vi "PolishVisionV4.vi"() -> (0 "Status":bool, 1 "Source CODE Robot":string, 3 "WorkPiece In Process":T1(plugin-control))   [LabVIEW 2015]
uses:
  <vilib>/userdefined/High Color/IMAQdx.ctl
  <vilib>/vision/driver/NI_Vision_Acquisition_Software.lvlib
  <vilib>/vision/NI_Vision_Development_Module.lvlib
panel:
  out "Edge Right Side":cluster{cluster{"Xrn":dbl, "Yrn":dbl}}[][](array[cluster])
  out "Edge Lefe Side":cluster{cluster{"Xln":dbl, "Yln":dbl}}[][](array[cluster])
  in  "WP Length":sgl=177.0
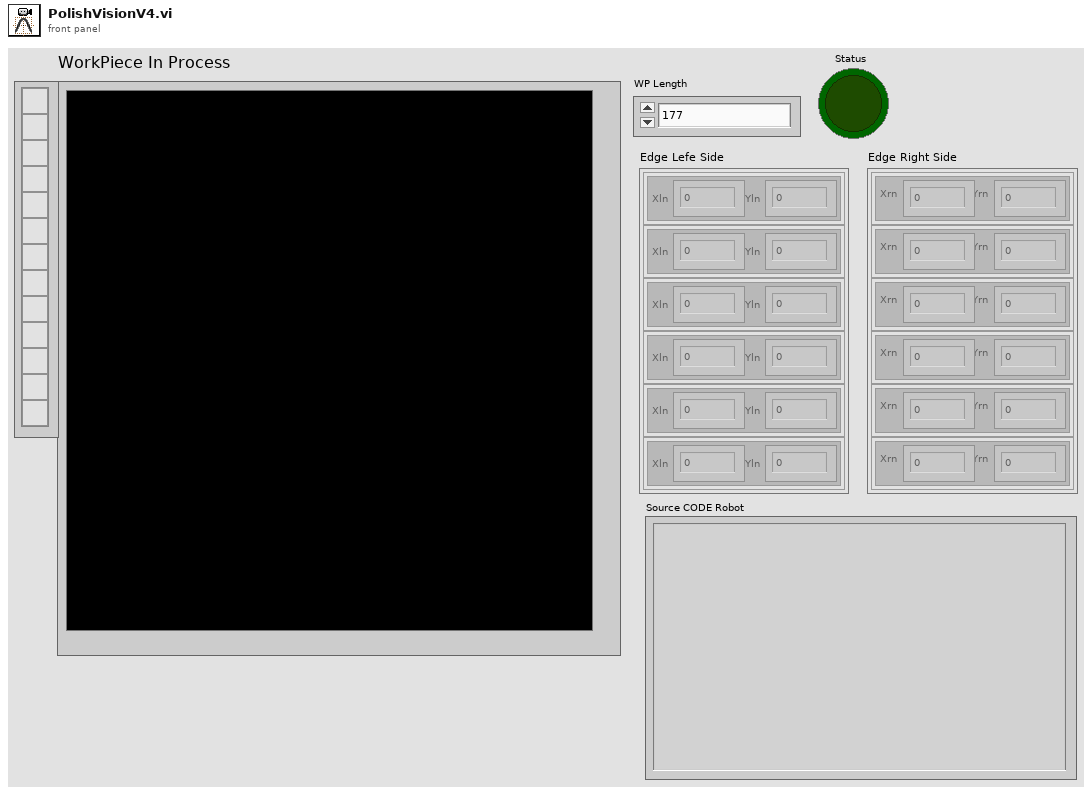
[diagram p1: front panel]
types:
  T1 = typedef "IMAQ Image.ctl" = refnum<image>
  T2 = typedef "IMAQdx.ctl" = refnum<k21>
  T3 = typedef "Image Type" = u32
  T4 = cluster{"Number of Matches Requested":i32, "Minimum Match Score":sgl, "Angle Ranges":cluster{"Start Angle":sgl, "End Angle":sgl}[]}
  T5 = cluster{"Global Rectangle":i32[], "Contours":cluster{"ID":enum32{"External", "Internal"}, "Type":u32, "Coordinates":i32[]}[]}
  T6 = cluster{"Origin Pixel":cluster{"X":sgl, "Y":sgl}, "X Axis Pixel":cluster{"X":sgl, "Y":sgl}, "Axis Reference":u32}
  T7 = cluster{"Position":cluster{"x":sgl, "y":sgl}, "Angle":sgl, "Scale":sgl, "Score":sgl, "Bounding Box":cluster{"x":sgl, "y":sgl}[]}[]
  T8 = cluster{"Feature":u32, "Points IDs":cluster{"GUID":string, "Index":i32}[]}[]
  T9 = cluster{"Matches (pixel)[0]":cluster{"Position":cluster{"x":sgl, "y":sgl}, "Angle":sgl, "Scale":sgl, "Score":sgl, "Bounding Box":cluster{"x":sgl, "y":sgl}[]}, "Matches (pixel)[1]":cluster{"Position":cluster{"x":sgl, "y":sgl}, "Angle":sgl, "Scale":sgl, "Score":sgl, "Bounding Box":cluster{"x":sgl, "y":sgl}[]}, "Matches (pixel)[2]":cluster{"Position":cluster{"x":sgl, "y":sgl}, "Angle":sgl, "Scale":sgl, "Score":sgl, "Bounding Box":cluster{"x":sgl, "y":sgl}[]}, "Matches (pixel)[3]":cluster{"Position":cluster{"x":sgl, "y":sgl}, "Angle":sgl, "Scale":sgl, "Score":sgl, "Bounding Box":cluster{"x":sgl, "y":sgl}[]}, "Matches (pixel)[4]":cluster{"Position":cluster{"x":sgl, "y":sgl}, "Angle":sgl, "Scale":sgl, "Score":sgl, "Bounding Box":cluster{"x":sgl, "y":sgl}[]}, "Matches (pixel)[5]":cluster{"Position":cluster{"x":sgl, "y":sgl}, "Angle":sgl, "Scale":sgl, "Score":sgl, "Bounding Box":cluster{"x":sgl, "y":sgl}[]}, "Matches (pixel)[6]":cluster{"Position":cluster{"x":sgl, "y":sgl}, "Angle":sgl, "Scale":sgl, "Score":sgl, "Bounding Box":cluster{"x":sgl, "y":sgl}[]}, "Matches (pixel)[7]":cluster{"Position":cluster{"x":sgl, "y":sgl}, "Angle":sgl, "Scale":sgl, "Score":sgl, "Bounding Box":cluster{"x":sgl, "y":sgl}[]}, "Matches (pixel)[8]":cluster{"Position":cluster{"x":sgl, "y":sgl}, "Angle":sgl, "Scale":sgl, "Score":sgl, "Bounding Box":cluster{"x":sgl, "y":sgl}[]}}
  T10 = cluster{"Results (Pixels)[0]":sgl, "Results (Pixels)[1]":sgl, "Results (Pixels)[2]":sgl, "Results (Pixels)[3]":sgl, "Results (Pixels)[4]":sgl, "Results (Pixels)[5]":sgl, "Results (Pixels)[6]":sgl, "Results (Pixels)[7]":sgl, "Results (Pixels)[8]":sgl}
  T11 = cluster{"Results (Pixels)[0]":sgl, "Results (Pixels)[1]":sgl}
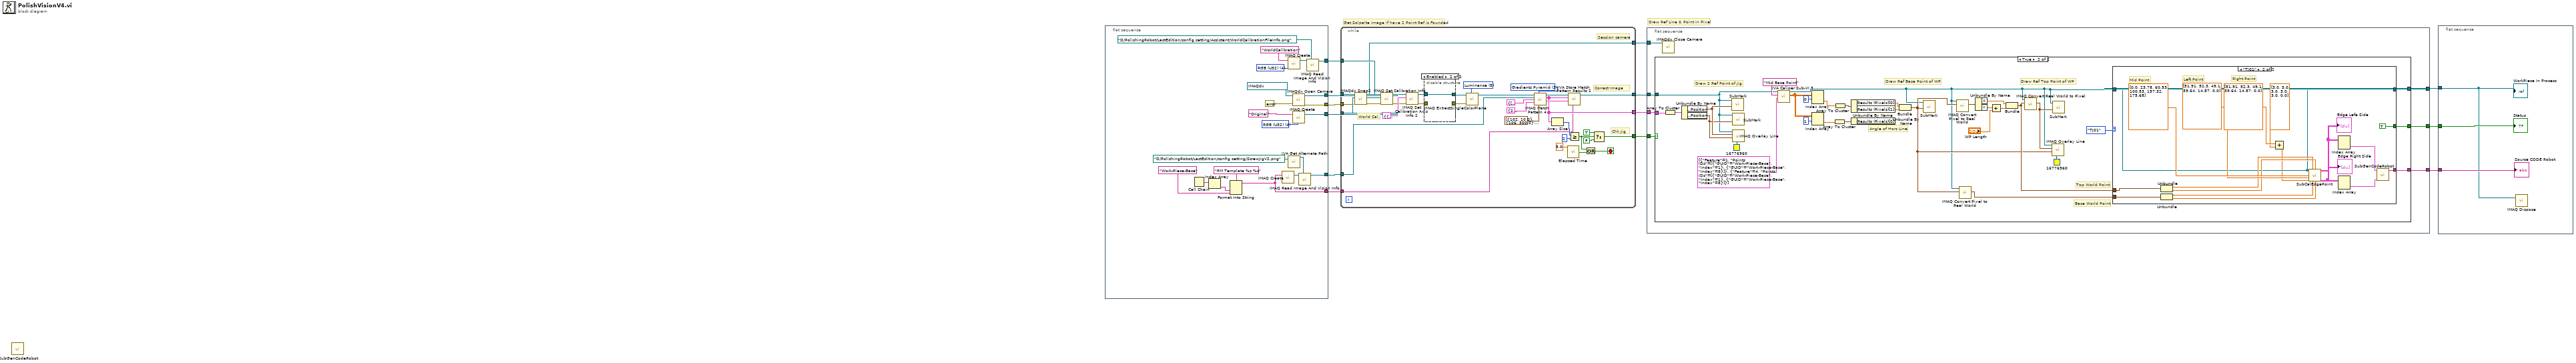
[diagram p0: block diagram]
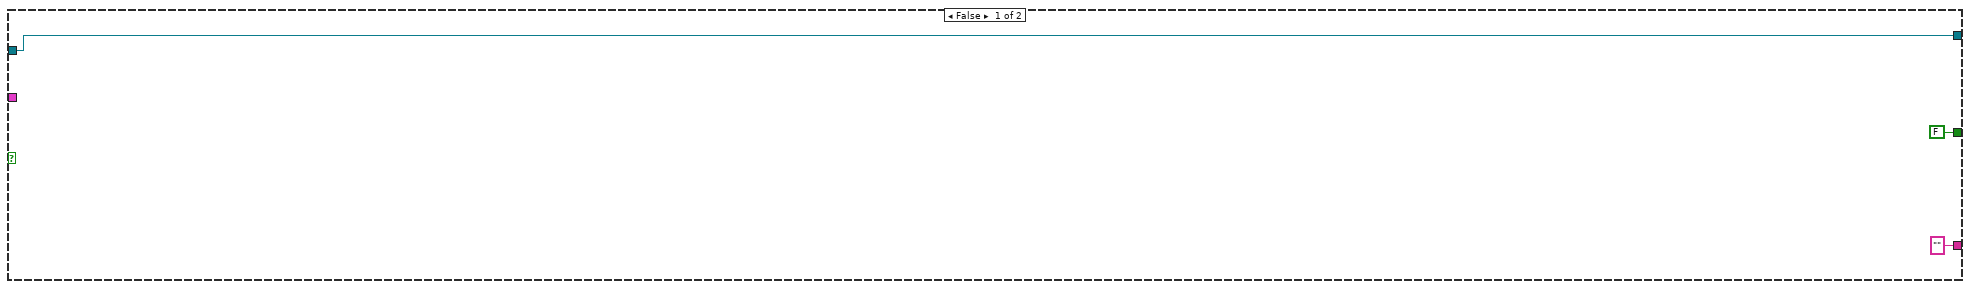
[diagram p2: hidden frame]
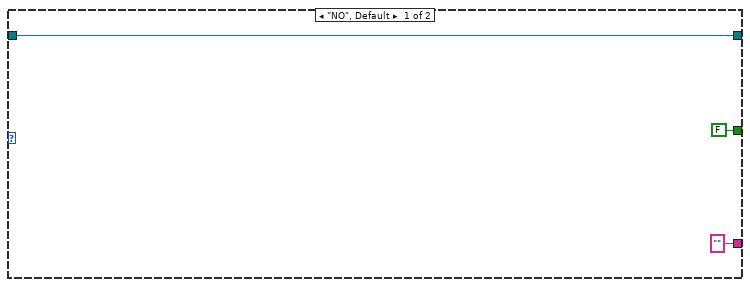
[diagram p3: hidden frame]
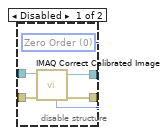
[diagram p4: hidden frame]
diagram:
  # "Draw Ref Line & Point in Pixel"
  # "Get Solpalte Image if have 2 Point Ref is Founded"
  n1 = call "SubGenCodeRobot.vi"() -> ()  [unwired: 11 in, 1 out]
  n2 = flat-sequence {
    tunnel: [w31] -> w13
    tunnel: [w30] -> w12
    tunnel: [w29] -> w10
    tunnel: [w23] -> w11
    tunnel: [w19] -> w9
    tunnel: [w14] -> w5
    frame #0 {
      w27 = T3 4 items=["Grayscale (U8)", "Grayscale (I16)", "Grayscale (SGL)", "Complex (CSG)", "RGB (U32)", "HSL (U32)", "RGB (U64)", "Grayscale (U16)"] ("Image Type")
      w32 = T3 4 items=["Grayscale (U8)", "Grayscale (I16)", "Grayscale (SGL)", "Complex (CSG)", "RGB (U32)", "HSL (U32)", "RGB (U64)", "Grayscale (U16)"] ("Image Type")
      n3 = Call Chain() -> (call chain=w17:string[])
      n4 = Index Array(array=w17) -> (element=w16:string)  [unwired: 1 in]
      n5 = Format Into String(format string="PM Template %s %s" ("Image Name"), w16, "Work-Piece-Base" ("Image Name")) -> (resulting string=w14:string)  [unwired: 2 in, 1 out]
      n6 = call "IMAQ Create"("Image Name"=w14) -> ("New Image"=w22:T1)  [unwired: 3 in, 2 out]
      n7 = call <vilib>:"IVA Get Alternate Path.vi"("Path In"=path "D:/PolishingRobot/LastEdition/config setting/ScrewJigV2.png" ("Template File Path")) -> ("Path Out"=w20:path)  [unwired: 10 out]
      n8 = call "IMAQ Create"("Image Name"="WorldCalibration", "Image Type"=w27) -> ("New Image"=w26:T1)  [unwired: 2 in, 2 out]
      n9 = call <vilib>:"IMAQdx Open Camera.vi"("error in"=errorcluster {"status"=FALSE, "code"=0, "source"=""}, "Session In"=T2 "RobotPolishCAM") -> ("error out"=w29:errorcluster, "Session Out"=w31:T2)  [unwired: 8 in]
      n10 = call "IMAQ Create"("Image Name"="Original", "Image Type"=w32) -> ("New Image"=w30:T1)  [unwired: 3 in, 1 out]
      n11 = call "IMAQ Read Image And Vision Info"("File Path"=w20, "Image"=w22) -> ("Image Out"=w19:T1)  [unwired: 2 in, 7 out]
      n12 = call "IMAQ Read Image And Vision Info"("File Path"=path "D:/PolishingRobot/LastEdition/config setting/Assistant/WorldCalibrationFileInfo.png", "Image"=w26) -> ("Image Out"=w23:T1)  [unwired: 2 in, 7 out]
    }
  }
  n13 = while {
    tunnel: w13 -> [w69]
    tunnel: w12 -> [w68]
    tunnel: w11 -> [w58]
    tunnel: w10 -> [w57]
    tunnel: [w55] -> w8
    tunnel: w9 -> [w47]
    tunnel: [w43] -> w6
    tunnel: [w42] -> w7
    tunnel: w5 -> [w38]
    tunnel: [w36] -> w4
    stop <- w60 stop-if-true
    w54 = 3 items=["All", "Low Discrepancy Sampling", "Grayscale Value Pyramid", "Gradients Pyramid"] ("Algorithm")
    w67 = 5 items=["Red", "Green", "Blue", "Hue", "Saturation", "Luminance", "Value", "Intensity"] ("Color Plane")
    # "Chk Jig"
    # "Correct Image"
    # "Session camera"
    # "World Cal."
    n14 = call <vilib>:"IMAQdx Snap2.vi"("error in"=w57, "Image In"=w68, "Session In"=w69) -> ("error out"=w56:errorcluster, "Image Out"=w59:T1, "Session Out"=w55:T2)  [unwired: 6 in]
    n15 = call "IMAQ Set Calibration Info"("error in (no error)"=w56, "Image Dst"=w59, "Image Src"=w58) -> ("error out"=w41:errorcluster, "Calibrated Image"=w65:T1)  [unwired: 1 in, 6 out]
    n16 = call-poly "IMAQ Set Calibration Axis Info 2"("error in (no error)"=w41, "Calibration Axis Info"=T6 {"Origin Pixel"={"X"=1113.64, "Y"=2715.63}, "X Axis Pixel"={"X"=1115.59, "Y"=2715.63}, "Axis Reference"=0}, "Calibration Template Image In"=w65) -> ("error out"=w40:errorcluster, "Calibration Template Image Out"=w64:T1)  [unwired: 7 out]
    n17 = disable-structure shown="Enabled" {
      disable-tunnel: w64 -> [w73 w75]
      disable-tunnel: [w72 w75] -> w63
      disable-tunnel: w40 -> [w71 _]
      disable-tunnel: [w70 _] -> w39
      frame Disabled {
        w74 = u32 0 items=["Zero Order", "Bi-Linear", "Quadratic", "Cubic Spline"] ("Interpolation Type")
        n18 = call "IMAQ Correct Calibrated Image"("Interpolation Type"=w74, "error in (no error)"=w71, "Image Src"=w73) -> ("error out"=w70:errorcluster, "Corrected Image"=w72:T1)  [unwired: 4 in, 3 out]
      }
      frame Enabled {
      }
    }
    n19 = call "IMAQ ExtractSingleColorPlane"("Color Plane"=w67, "error in (no error)"=w39, "Image Src"=w63) -> ("Image Dst Out"=w48:T1)  [unwired: 7 in, 1 out]
    n20 = call "IMAQ Match Pattern 4"("Image"=w48, "Algorithm"=w54, "Template Image"=w47, "ROI Descriptor"=T5 {"Global Rectangle"=[500, 650, 1500, 800], "Contours"=[{"ID"=enum."External", "Type"=12, "Coordinates"=[500, 650, 1500, 800, 0]}]}, "Parameters"=T4 {"Number of Matches Requested"=2, "Minimum Match Score"=500.0, "Angle Ranges"=[]}, "Advanced Options"=cluster{"Item":u16, "Value":dbl}[] [{"Item"=102, "Value"=10.0}, {"Item"=106, "Value"=300.0}, {"Item"=107, "Value"=0.0}, {"Item"=108, "Value"=6.0}, {"Item"=109, "Value"=1.0}, {"Item"=111, "Value"=20.0}, {"Item"=112, "Value"=10.0}, {"Item"=113, "Value"=20.0}, {"Item"=103, "Value"=1.0}, {"Item"=100, "Value"=1.0}]) -> ("Image (duplicate)"=w37:T1, "Matches (pixel)"=w42:T7, "Matches (real-world)"=w35:T7)  [unwired: 5 in, 2 out]
    n21 = Array Size(array=w42) -> (size(s)=w49:i32)
    n22 = call "Elapsed Time"("Time Target (s)"=5.0) -> ("Time has Elapsed"=w61:bool)  [unwired: 11 in, 7 out]
    n23 = call <vilib>:"IVA Store Match Pattern Results 2.vi"("Step Name"=w38, "Matches (real-world)"=w35, "Matches (pixel)"=w42, "Image in"=w37) -> ("Image dup"=w36:T1)  [unwired: 2 in, 5 out]
    n24 = Greater Or Equal?(x=w49, y=2) -> (x >= y?=w46:bool)
    n25 = Or(x=w46, y=w61) -> (x .or. y?=w60:bool)
    n26 = Select(t=TRUE, s=w46, f=FALSE) -> (s? t:f=w43:bool)
  }
  n27 = flat-sequence {
    tunnel: w8 -> [w82]
    tunnel: w7 -> [w81]
    tunnel: w6 -> [w80]
    tunnel: w4 -> [w79]
    tunnel: [w78] -> w3
    tunnel: [w77] -> w2
    tunnel: [w76] -> w1
    frame #0 {
      n28 = case shown="True" w80 {
        tunnel: w81 -> [_ w113]
        tunnel: w79 -> [w85 w105]
        tunnel: [w85 w88] -> w78
        tunnel: ["" ("Source CODE Robot") w87] -> w77
        tunnel: [FALSE w86] -> w76
        frame False {
        }
        frame True {
          # "Base World Point"
          # "Top World Point"
          # "Draw Ref Top Point of WP"
          # "Angle of Horz Line"
          # "Draw Ref Base Point of WP"
          # "Draw 2 Ref Point of Jig"
          n29 = Array To Cluster(array=w113) -> (cluster=w117:T9)
          n30 = Unbundle By Name(w117) -> ("Matches (pixel)[0].Position"=w115:cluster{"x":sgl, "y":sgl}, "Matches (pixel)[1].Position"=w114:cluster{"x":sgl, "y":sgl})
          n31 = call "SubMark.vi"("Refnum in"=w105, "Position Pixel"=w115) -> ()  [unwired: 8 in]
          n32 = call "SubMark.vi"("Refnum in"=w105, "Position Pixel"=w114) -> ()  [unwired: 8 in]
          n33 = call "IMAQ Overlay Line"("Color"=u32 16776960, "End Point"=w114, "Start Point"=w115, "Image"=w105) -> ()  [unwired: 6 in, 2 out]
          n34 = call <vilib>:"IVA Caliper Sub-VI 3.vi"("Parameters"=T8 [{"Feature"=1, "Points IDs"=[{"GUID"="Work-Piece-Base", "Index"=1}, {"GUID"="Work-Piece-Base", "Index"=8}]}, {"Feature"=4, "Points IDs"=[{"GUID"="Work-Piece-Base", "Index"=1}, {"GUID"="Work-Piece-Base", "Index"=8}]}], "Step Name"="Mid Base Point", "Image In"=w105) -> ("Results (Pixels)"=w103:sgl[][], "Image Out"=w90:T1)  [unwired: 2 in, 5 out]
          n35 = Index Array(array=w103, index (row)=0) -> (element=w110:sgl[])  [unwired: 1 in]
          n36 = Index Array(array=w103, index (row)=1) -> (element=w102:sgl[])  [unwired: 1 in]
          n37 = Array To Cluster(array=w102) -> (cluster=w101:T10)
          n38 = Array To Cluster(array=w110) -> (cluster=w108:T10)
          n39 = Unbundle By Name(w108) -> ("Results (Pixels)[0]"=w107:sgl, "Results (Pixels)[1]"=w106:sgl)
          n40 = Unbundle By Name(w101) -> ()  [unwired: 1 out]
          n41 = Bundle("Results (Pixels)[0]"=w107, "Results (Pixels)[1]"=w106) -> (w91:T11)  [unwired: 1 in]
          n42 = call "SubMark.vi"("Refnum in"=w90, "Position Pixel"=w91) -> ()  [unwired: 8 in]
          n43 = call "IMAQ Convert Pixel to Real World"("Pixel Coordinates"=w91, "Calibrated Image"=w90) -> ("Real World Coordinates"=w98:cluster{"X":sgl, "Y":sgl})  [unwired: 4 in, 5 out]
          n44 = call "IMAQ Convert Pixel to Real World"("Pixel Coordinates"=w91, "Calibrated Image"=w90) -> ("Real World Coordinates"=w89:cluster{"X":sgl, "Y":sgl})  [unwired: 4 in, 5 out]
          n45 = Unbundle By Name(w98) -> ("X"=w96:sgl, "Y"=w99:sgl)
          n46 = Add(x=w99, y="WP Length") -> (x+y=w97:sgl)
          n47 = Bundle("X"=w96, w97) -> (w92:cluster{"X":sgl, sgl})  [unwired: 1 in]
          n48 = call "IMAQ Convert Real World to Pixel"("Real World Coordinates"=w92, "Calibrated Image"=w90) -> ("Pixel Coordinates"=w95:cluster{"X":sgl, "Y":sgl})  [unwired: 4 in, 5 out]
          n49 = call "IMAQ Overlay Line"("Color"=u32 16776960, "End Point"=w91, "Start Point"=w95, "Image"=w90) -> ()  [unwired: 6 in, 2 out]
          n50 = call "SubMark.vi"("Refnum in"=w90, "Position Pixel"=w95) -> ()  [unwired: 8 in]
          n51 = case shown="\"TJ01\"" enum16{"NO", "TJ02", "TJ01"}."TJ01" {
            tunnel: w90 -> [w120 w130]
            tunnel: w92 -> [_ w135]
            tunnel: w89 -> [_ w136]
            tunnel: [w120 w130] -> w88
            tunnel: ["" ("Source CODE Robot") w122] -> w87
            tunnel: [FALSE TRUE] -> w86
            frame "NO", Default {
            }
            frame "TJ01" {
              # "Right Point"
              # "Left Point"
              # "Mid Point"
              n52 = Unbundle(w135) -> ("X"=w134:sgl, w133:sgl)
              n53 = Unbundle(w136) -> ("X"=w132:sgl, "Y"=w131:sgl)
              n54 = Add(x=dbl[] [51.91, 52.3, 49.1, 39.64, 14.87, 0.0] ("Mid Point"), y=dbl[] [3.0, 3.0, 3.0, 3.0, 3.0, 0.0]) -> (x+y=w127:dbl[])
              n55 = call "SubCalEdgePoint.vi"("Image dup"=w130, "Mid Point Top World X"=w134, "Mid Point Top World Y"=w133, "Mid Point"=dbl[] [0.0, 23.78, 60.53, 100.53, 157.32, 175.68], "Left Point"=dbl[] [51.91, 52.3, 49.1, 39.64, 14.87, 0.0] ("Mid Point"), "Right Point"=w127, "Mid Point Base World X"=w132, "Mid Point Base World Y"=w131) -> ("Edge Lefe Side"=w126:cluster{cluster{"Xln":dbl, "Yln":dbl}}[][], "Edge Right Side"=w123:cluster{cluster{"Xrn":dbl, "Yrn":dbl}}[][])  [unwired: 6 in]
              "Edge Lefe Side" <- w126
              "Edge Right Side" <- w123
              n56 = Index Array(array=w126) -> (element=w125:cluster{cluster{"Xln":dbl, "Yln":dbl}}[])  [unwired: 2 in]
              n57 = Index Array(array=w123) -> (element=w124:cluster{cluster{"Xrn":dbl, "Yrn":dbl}}[])  [unwired: 2 in]
              n58 = call "SubGenCodeRobot.vi"("Edge Right Side"=w124, "Edge Left Side"=w125) -> ("Source CODE Robot"=w122:string)  [unwired: 9 in]
            }
          }
        }
      }
      n59 = call <vilib>:"IMAQdx Close Camera.vi"("Session In"=w82) -> ()  [unwired: 10 in, 1 out]
    }
  }
  n60 = flat-sequence {
    tunnel: w3 -> [w139]
    tunnel: w2 -> [w141]
    tunnel: w1 -> [w140]
    frame #0 {
      n61 = call "IMAQ Dispose"("Image"=w139) -> ()  [unwired: 5 in, 1 out]
      "WorkPiece In Process" <- w139
      "Source CODE Robot" <- w141
      "Status" <- w140
    }
  }
